vi "SavedStatusUpdate.vi"(7 "Options":enum16{"Unsaved", "Saved"}(ring), 8 "error in (no error)":errorcluster, 11 "UI control refnums":T1) -> (0 "error out":errorcluster)   [LabVIEW 2012]
doc: "SciScan 1.2 160622"
uses:
  Custom Controls and Typedefs/Macro_MD_UI Control Refnums.ctl
  Custom Controls and Typedefs/Delete Button.ctl
  Custom Controls and Typedefs/Edit Button.ctl
  Custom Controls and Typedefs/Timing Estimate Cluster.ctl
  CommonResource VIs/Timing/Timing Indicator.ctl
  Custom Controls and Typedefs/Load from PSM Button.ctl
panel:
  # "(hh:mm:ss)"
  # "(hh:mm:ss)"
  # "(hh:mm:ss)"
  # "(hh:mm:ss)"
  # "(hh:mm:ss)"
  # "(hh:mm:ss)"
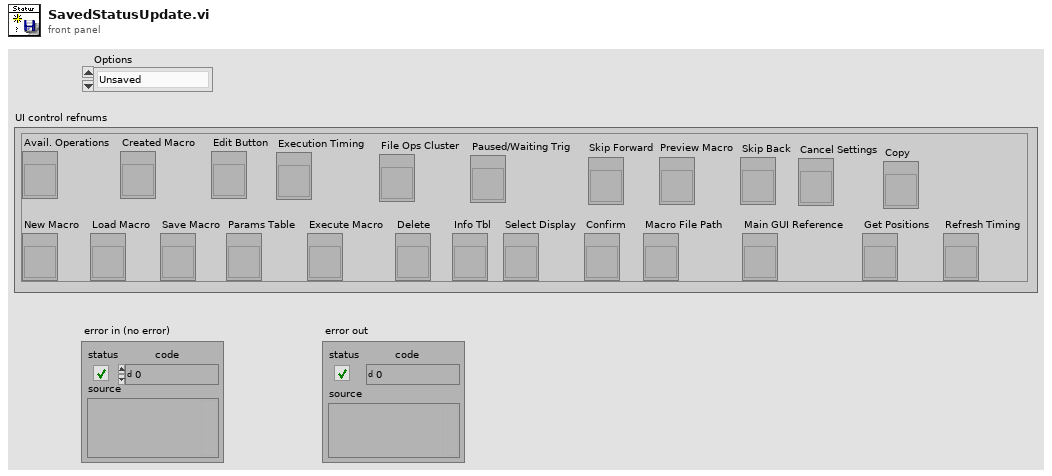
[diagram p1: front panel]
types:
  T1 = typedef "Macro_MD_UI Control Refnums.ctl" = cluster{"Avail. Operations":refnum<vi>, "Created Macro":refnum<vi>, "Load Macro":refnum<vi>, "Save Macro":refnum<vi>, "Params Table":refnum<vi>, "Delete":refnum<vi>, "Edit Button":refnum<vi>, "Execute Macro":refnum<vi>, "Info Tbl":refnum<vi>, "Execution Timing":refnum<vi>, "Select Display":refnum<vi>, "File Ops Cluster":refnum<vi>, "Paused/Waiting Trig":refnum<vi>, "Confirm":refnum<vi>, "New Macro":refnum<vi>, "Preview Macro":refnum<vi>, "Skip Forward":refnum<vi>, "Skip Back":refnum<vi>, "Macro File Path":refnum<vi>, "Main GUI Reference":refnum<vi>, "Cancel Settings":refnum<vi>, "Get Positions":refnum<vi>, "Copy":refnum<vi>, "Refresh Timing":refnum<vi>}
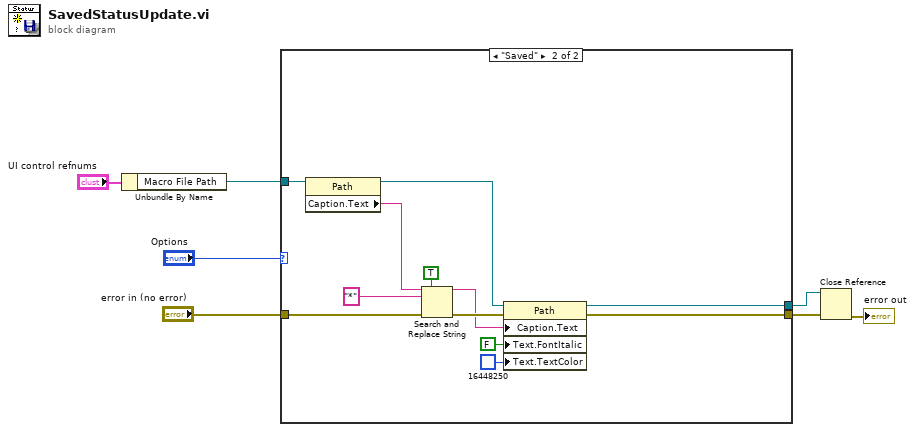
[diagram p0: block diagram]
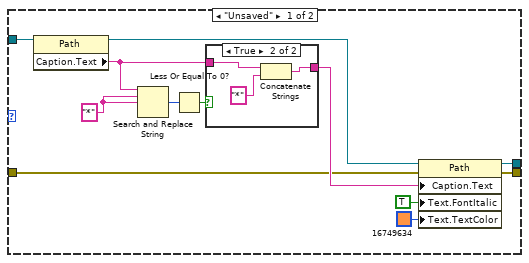
[diagram p2: hidden frame]
diagram:
  n1 = Unbundle By Name("UI control refnums") -> ("Macro File Path"=w4:refnum<vi>)
  n2 = case shown="\"Saved\"" "Options" {
    tunnel: "error in (no error)" -> [w14 w29]
    tunnel: w4 -> [w17 w34]
    tunnel: [w16 w33] -> w3
    tunnel: [w15 w32] -> w2
    frame "Unsaved" {
      w12 = "*" ("string")
      n3 = property class="Path"(reference=w17) -> (reference out=w18:refnum<vi>, "Caption.Text"=w13:string)  [unwired: 1 in, 1 out]
      n4 = Search and Replace String(input string=w13, search string=w12, replace string=w12) -> (number of replacements=w11:i32)  [unwired: 5 in, 3 out]
      n5 = Less Or Equal To 0?(x=w11) -> (x <= 0?=w10:bool)
      n6 = case shown="True" w10 {
        tunnel: [w20 w22] -> w19
        tunnel: w13 -> [w20 w21]
        frame False {
        }
        frame True {
          n7 = Concatenate Strings(w21, "*" ("string")) -> (w22:string)
        }
      }
      n8 = property class="Path"(reference=w18, error in=w14, "Caption.Text"=w19, "Text.FontItalic"=TRUE ("Path Text.Font:Italic"), "Text.TextColor"=u32 16749634) -> (reference out=w15:refnum<vi>, error out=w16:errorcluster)
    }
    frame "Saved" {
      n9 = property class="Path"(reference=w34) -> (reference out=w35:refnum<vi>, "Caption.Text"=w31:string)  [unwired: 1 in, 1 out]
      n10 = Search and Replace String(replace all?=TRUE ("replace all? (F)"), input string=w31, search string="*" ("string"), error in=w29) -> (result string=w27:string, error out=w28:errorcluster)  [unwired: 4 in, 2 out]
      n11 = property class="Path"(reference=w35, error in=w28, "Caption.Text"=w27, "Text.FontItalic"=FALSE ("Path Text.Font:Italic"), "Text.TextColor"=u32 16448250) -> (reference out=w32:refnum<vi>, error out=w33:errorcluster)
    }
  }
  n12 = Close Reference(reference=w2, error in (no error)=w3) -> (error out=→"error out":errorcluster)
